vi "LL_BuildElementPath_String.vi"(10 "Name":string, 11 "parent Name":string) -> (3 "full name":string)   [LabVIEW 2017, in "TOML.lvlib"]
uses:
  TOML.lvlib
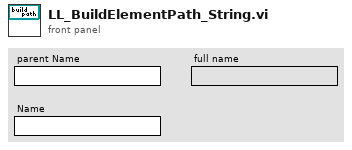
[diagram p1: front panel]
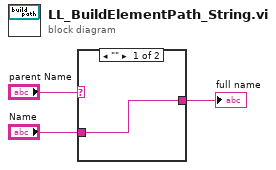
[diagram p0: block diagram]
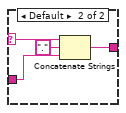
[diagram p2: hidden frame]
diagram:
  n1 = case shown="\"\"" "parent Name" {
    selector: "parent Name" -> [_ w5]
    tunnel: [w4 w7] -> w3
    tunnel: "Name" -> [w4 w6]
    frame "" {
    }
    frame Default {
      n2 = Concatenate Strings(w5, "." ("string"), w6) -> (w7:string)
    }
  }
  "full name" <- w3
